vi "ma_DesignIIRFilterCoeff.vi"(4 "Optional Filter Specifications":T3 {"PB Gain" format="%0.2f"; "SB Gain" format="%0.2f"; "Lower SB" format="%0.2p"; "Upper SB" format="%0.2f"; "Lower PB" format="%0.2p"; "Upper PB" format="%0.2f"}, 6 "Filter specifications":T4={"Topology"=enum."Bessel", "Type"=enum."Lowpass", "Order"=16340, "Lower Fc"=92.0, "Upper Fc"=0.0, "PB Ripple"=0.0, "SB Attenuation"=0.0} {"PB Ripple" format="%0.2f"; "Lower Fc" format="%0.2p"; "SB Attenuation" format="%0.2f"; "Upper Fc" format="%0.2p"}, 7 "filter structure option":T1=10 items=["IIR 2nd Order"=0, "IIR 4th Order"=1, "Auto Select"=10], 8 "error in (no error)":errorcluster, 10 "Sampling Frequency":dbl format="%0.2f") -> (0 "error out":errorcluster, 2 "Filter Information":T2 {"phase H(w)"."df" format="%0.2f"; "phase H(w)"."f0" format="%0.2f"; "phase H(w)"."Phase H(w)" format="%0.2f"; "magnitude H(w)"."df" format="%0.2f"; "magnitude H(w)"."f0" format="%0.2f"; "magnitude H(w)"."Mag H(w)" format="%0.2f"}, 3 "IIR Filter Cluster":T5 {"Forward Coefficients" format="%0.2f"; "Reverse Coefficients" format="%0.2f"})   [LabVIEW 2020, in "NI_MAPro.lvlib"]
uses:
  NI_MAPro.lvlib
  Filter Structure Type.ctl
  NI_AALBase.lvlib
  NI_MABase.lvlib
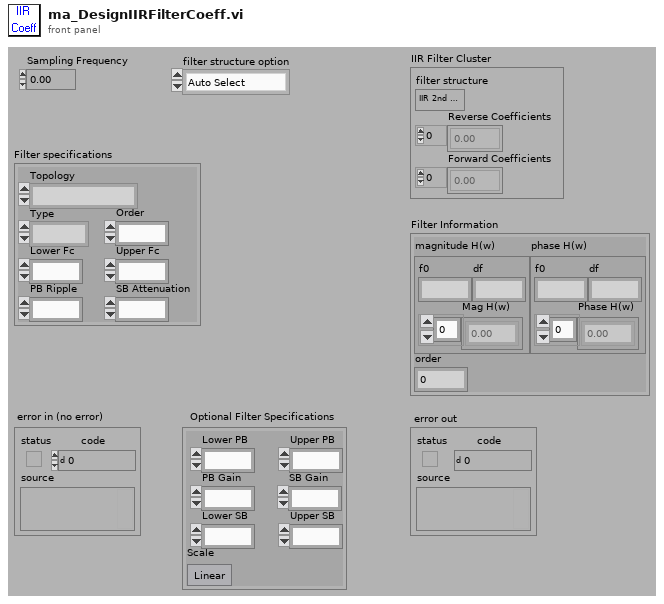
[diagram p1: front panel]
types:
  T1 = typedef "NI_AALBase.lvlib/Filter Structure Type.ctl" = u16
  T2 = cluster{"magnitude H(w)":cluster{"f0":dbl, "df":dbl, "Mag H(w)":dbl[]}, "phase H(w)":cluster{"f0":dbl, "df":dbl, "Phase H(w)":dbl[]}, "order":i32}
  T3 = cluster{"Lower PB":dbl, "Upper PB":dbl, "Lower SB":dbl, "Upper SB":dbl, "PB Gain":dbl, "SB Gain":dbl, "Scale":bool}
  T4 = cluster{"Topology":enum16{"Off", "Butterworth", "Chebyshev", "Inverse Chebyshev", "Elliptic", "Bessel"}, "Type":enum16{"Lowpass", "Highpass", "Bandpass", "Bandstop"}, "Order":i32, "Lower Fc":dbl, "Upper Fc":dbl, "PB Ripple":dbl, "SB Attenuation":dbl}
  T5 = cluster{"filter structure":enum32{"IIR 2nd Order", "IIR 4th Order"}, "Reverse Coefficients":dbl[], "Forward Coefficients":dbl[]}
  T6 = enum16{"Off", "Butterworth", "Chebyshev", "Inverse Chebyshev", "Elliptic", "Bessel"}
  T7 = enum16{"Lowpass", "Highpass", "Bandpass", "Bandstop"}
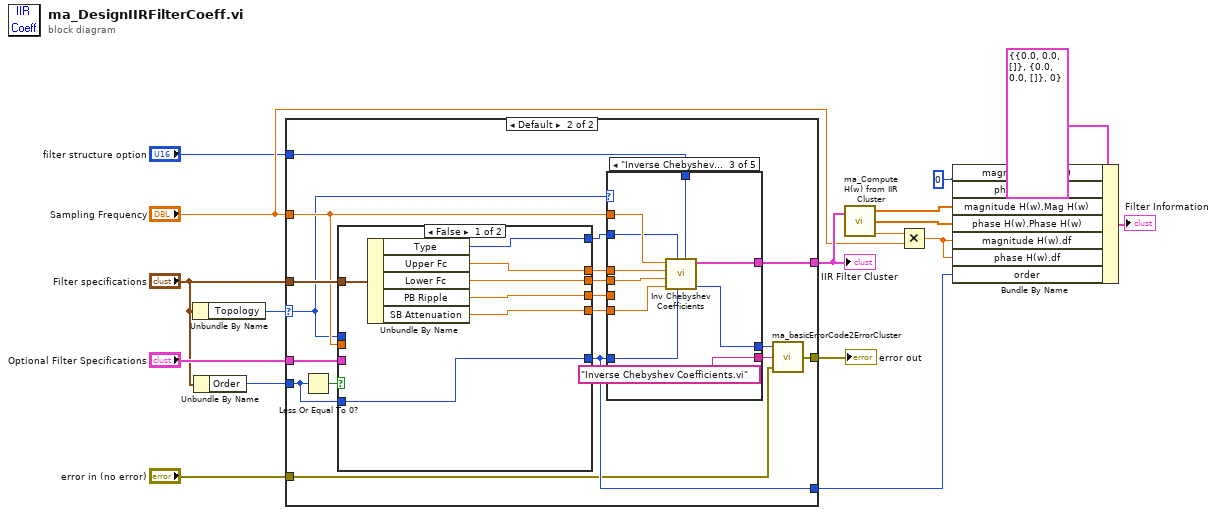
[diagram p0: block diagram]
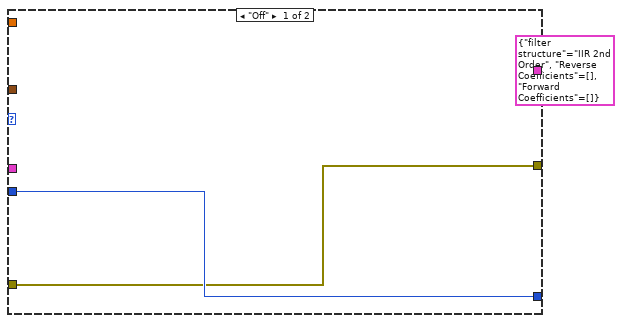
[diagram p2: hidden frame]
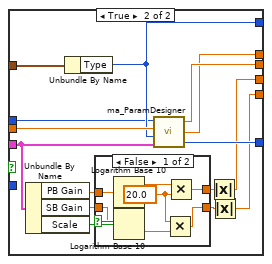
[diagram p3: hidden frame]
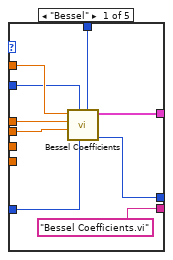
[diagram p5: hidden frame]
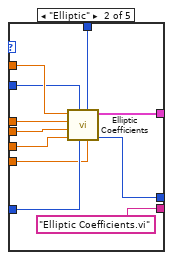
[diagram p6: hidden frame]
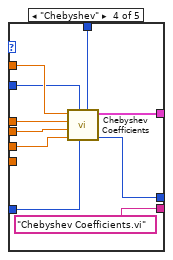
[diagram p7: hidden frame]
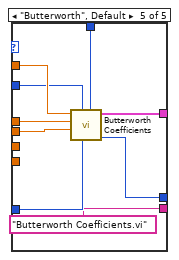
[diagram p8: hidden frame]
diagram:
  w4 = 0
  n1 = Unbundle By Name("Filter specifications") -> ("Topology"=w14:T6)
  n2 = Unbundle By Name("Filter specifications") -> ("Order"=w16:i32)
  n3 = case shown="Default" w14 {
    selector: w14 -> [_ w29]
    tunnel: [w19 w25] -> w13
    tunnel: "Optional Filter Specifications" -> [_ w33]
    tunnel: w16 -> [w20 w26]
    tunnel: "Filter specifications" -> [_ w32]
    tunnel: [T5 {"filter structure"=enum."IIR 2nd Order", "Reverse Coefficients"=[], "Forward Coefficients"=[]} ("IIR Filter Cluster") w31] -> w12
    tunnel: "Sampling Frequency" -> [_ w30]
    tunnel: [w20 w28] -> w7
    tunnel: "error in (no error)" -> [w19 w24]
    tunnel: "filter structure option" -> [_ w21]
    frame "Off" {
    }
    frame Default {
      n4 = Less Or Equal To 0?(x=w26) -> (x <= 0?=w27:bool)
      n5 = case shown="False" w27 {
        tunnel: w32 -> [w45 w60]
        tunnel: w30 -> [_ w59]
        tunnel: [w40 w58] -> w38
        tunnel: [w44 w55] -> w37
        tunnel: [w43 w56] -> w36
        tunnel: [w42 w47] -> w35
        tunnel: [w41 w46] -> w34
        tunnel: w33 -> [_ w53]
        tunnel: [w39 w57] -> w28
        tunnel: w29 -> [_ w54]
        tunnel: w26 -> [w39 _]
        frame False {
          n6 = Unbundle By Name(w45) -> ("Type"=w40:T7, "Upper Fc"=w44:dbl, "Lower Fc"=w43:dbl, "PB Ripple"=w42:dbl, "SB Attenuation"=w41:dbl)
        }
        frame True {
          n7 = Unbundle By Name(w53) -> ("PB Gain"=w52:dbl, "SB Gain"=w51:dbl, "Scale"=w48:bool)
          n8 = Unbundle By Name(w60) -> ("Type"=w58:T7)
          n9 = case shown="False" w48 {
            tunnel: w52 -> [w67 w68]
            tunnel: w51 -> [w66 w69]
            tunnel: [w62 w69] -> w50
            tunnel: [w61 w68] -> w49
            frame False {
              w63 = 20.0 ("y")
              n10 = Logarithm Base 10(1:w67) -> (0:w64:dbl)
              n11 = Logarithm Base 10(1:w66) -> (0:w65:dbl)
              n12 = Multiply(x=w63, y=w65) -> (x*y=w62:dbl)
              n13 = Multiply(x=w64, y=w63) -> (x*y=w61:dbl)
            }
            frame True {
            }
          }
          n14 = call "ma_ParamDesigner.vi"("Desired Filter Specifications"=w53, "Filter type"=w58, "Sampling Frequency"=w59, "Filter topology"=w54) -> ("filter order"=w57:i32, "fh"=w55:dbl, "fl"=w56:dbl)
          n15 = Absolute Value(x=w49) -> (abs(x)=w47:dbl)
          n16 = Absolute Value(x=w50) -> (abs(x)=w46:dbl)
        }
      }
      n17 = case shown="\"Inverse Chebyshev\"" w29 {
        tunnel: w28 -> [w78 w89 w99 w109 w113]
        tunnel: w30 -> [w77 w88 w98 w108 w118]
        tunnel: w38 -> [w76 w87 w97 w107 w117]
        tunnel: [w75 w86 w96 w106 w116] -> w31
        tunnel: [w72 w81 w92 w102 w112] -> w23
        tunnel: w37 -> [w74 w85 w95 w105 w115]
        tunnel: w36 -> [w73 w84 w94 w104 w114]
        tunnel: w35 -> [_ w83 _ w103 _]
        tunnel: w34 -> [_ w82 w93 _ _]
        tunnel: ["Bessel Coefficients.vi" "Elliptic Coefficients.vi" "Inverse Chebyshev Coefficients.vi" "Chebyshev Coefficients.vi" "Butterworth Coefficients.vi"] -> w22
        tunnel: w21 -> [w70 w79 w90 w100 w110]
        frame "Bessel" {
          n18 = call "Bessel Coefficients.vi"("filter structure option"=w70, "order"=w78, "filter type"=w76, "low cutoff freq: fl"=w73, "high cutoff freq: fh"=w74, "sampling freq: fs"=w77) -> ("error"=w72:i32, "IIR Filter Cluster"=w75:T5)  [unwired: 4 in]
        }
        frame "Elliptic" {
          n19 = call "Elliptic Coefficients.vi"("stopband attenuation (dB)"=w82, "filter structure option"=w79, "order"=w89, "filter type"=w87, "passband ripple (dB)"=w83, "low cutoff freq: fl"=w84, "high cutoff freq: fh"=w85, "sampling freq: fs"=w88) -> ("error"=w81:i32, "IIR Filter Cluster"=w86:T5)  [unwired: 2 in]
        }
        frame "Inverse Chebyshev" {
          n20 = call "Inv Chebyshev Coefficients.vi"("filter structure option"=w90, "order"=w99, "filter type"=w97, "attenuation (dB)"=w93, "low cutoff freq: fl"=w94, "high cutoff freq: fh"=w95, "sampling freq: fs"=w98) -> ("error"=w92:i32, "IIR Filter Cluster"=w96:T5)  [unwired: 3 in]
        }
        frame "Chebyshev" {
          n21 = call "Chebyshev Coefficients.vi"("filter structure option"=w100, "order"=w109, "filter type"=w107, "ripple(dB)"=w103, "low cutoff freq: fl"=w104, "high cutoff freq: fh"=w105, "sampling freq: fs"=w108) -> ("error"=w102:i32, "IIR Filter Cluster"=w106:T5)  [unwired: 3 in]
        }
        frame "Butterworth", Default {
          n22 = call "Butterworth Coefficients.vi"("filter structure option"=w110, "order"=w113, "filter type"=w117, "low cutoff freq: fl"=w114, "high cutoff freq: fh"=w115, "sampling freq: fs"=w118) -> ("error"=w112:i32, "IIR Filter Cluster"=w116:T5)  [unwired: 4 in]
        }
      }
      n23 = call "ma_basicErrorCode2ErrorCluster.vi"("error in (no error)"=w24, "subVI name"=w22, "Error Code"=w23) -> ("error out"=w25:errorcluster)
    }
  }
  "IIR Filter Cluster" <- w12
  "error out" <- w13
  n24 = call "ma_Compute H(w) from IIR Cluster.vi"("IIR Filter Cluster"=w12) -> ("Mag H(w)"=w8:dbl[], "Phase H(w)"=w3:dbl[], "df"=w11:dbl)  [unwired: 1 in]
  n25 = Multiply(x=w11, y="Sampling Frequency") -> (x*y=w5:dbl)
  n26 = Bundle By Name(cluster=T2 {"magnitude H(w)"={"f0"=0.0, "df"=0.0, "Mag H(w)"=[]}, "phase H(w)"={"f0"=0.0, "df"=0.0, "Phase H(w)"=[]}, "order"=0} ("Filter Information"), "magnitude H(w).f0"=w4, "phase H(w).f0"=w4, "magnitude H(w).Mag H(w)"=w8, "phase H(w).Phase H(w)"=w3, "magnitude H(w).df"=w5, "phase H(w).df"=w5, "order"=w7) -> (→"Filter Information":T2)
